vi "Database.Main-GetTime.vi"() -> (0 "TS":timestamp)   [LabVIEW 2016]
doc: "Go to DB->WriteStationValues action\nReturn boolean flag to show if data was saved to DB successfully\n\nWabco 2017 All right reserved\nAuthor: maciej.szupienko@wabco-auto.com"
uses:
  Database.Global.vi
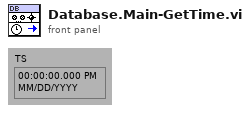
[diagram p1: front panel]
types:
  T1 = typedef "Database.Main.Data.Status.ctl" = cluster{"Run":bool, "Handle":i32, "ConnTS":timestamp, "DbTime":timestamp, "DbTimeCode":dbl, "DbTimeOffset":dbl}
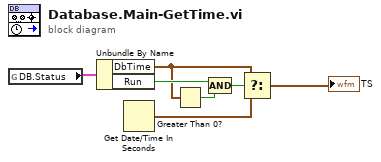
[diagram p0: block diagram]
diagram:
  n1 = global read "Database.Global.vi" "DB.Status"() -> (w7:T1)
  n2 = Unbundle By Name(w7) -> ("DbTime"=w3:timestamp, "Run"=w6:bool)
  n3 = Get Date/Time In Seconds() -> (seconds since 1Jan1904=w5:timestamp)
  n4 = Greater Than 0?(x=w3) -> (x > 0?=w1:bool)
  n5 = Compound Arithmetic op=AND(w6, w1) -> (w2:bool)
  n6 = Select(t=w3, s=w2, f=w5) -> (s? t:f=→"TS":timestamp)
